vi "VoltageToResistance.vi"(1 "Reference Resistance (ohms)":dbl, 2 "Circuit Total Voltage (V)":dbl, 3 "Voltage Measured":dbl) -> (0 "Resistance Measured (ohms)":dbl)   [LabVIEW 2020]
panel:
  # "Returns the Resistance"
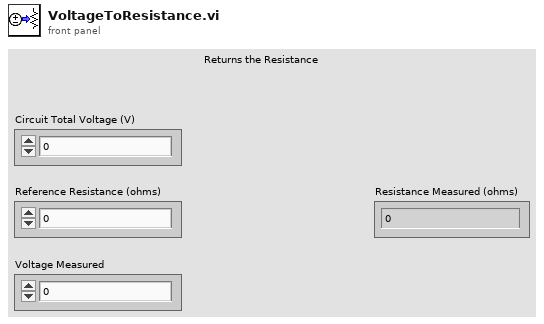
[diagram p1: front panel]
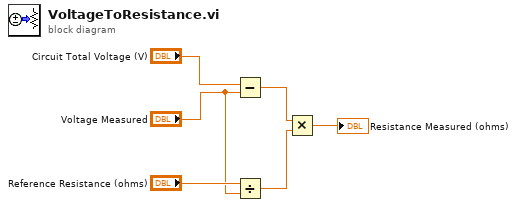
[diagram p0: block diagram]
diagram:
  n1 = Subtract(x="Circuit Total Voltage (V)", y="Voltage Measured") -> (x-y=w4:dbl)
  n2 = Divide(x="Reference Resistance (ohms)", y="Voltage Measured") -> (x/y=w5:dbl)
  n3 = Multiply(x=w4, y=w5) -> (x*y=→"Resistance Measured (ohms)":dbl)
